vi "servertest.vi"() -> ()   [LabVIEW 2017]
uses:
  <vilib>/httpClient/ClientHandle.ctl
  <vilib>/httpClient/POSTBuffer.vi
  <vilib>/httpClient/LabVIEWHTTPClient.lvlib
panel:
  out "temp":i32
  out "element":T1
  out "value 2":T2
  in  "?":T3
  in  "url":string="getTC"
  out "body":string
  out "headers":string
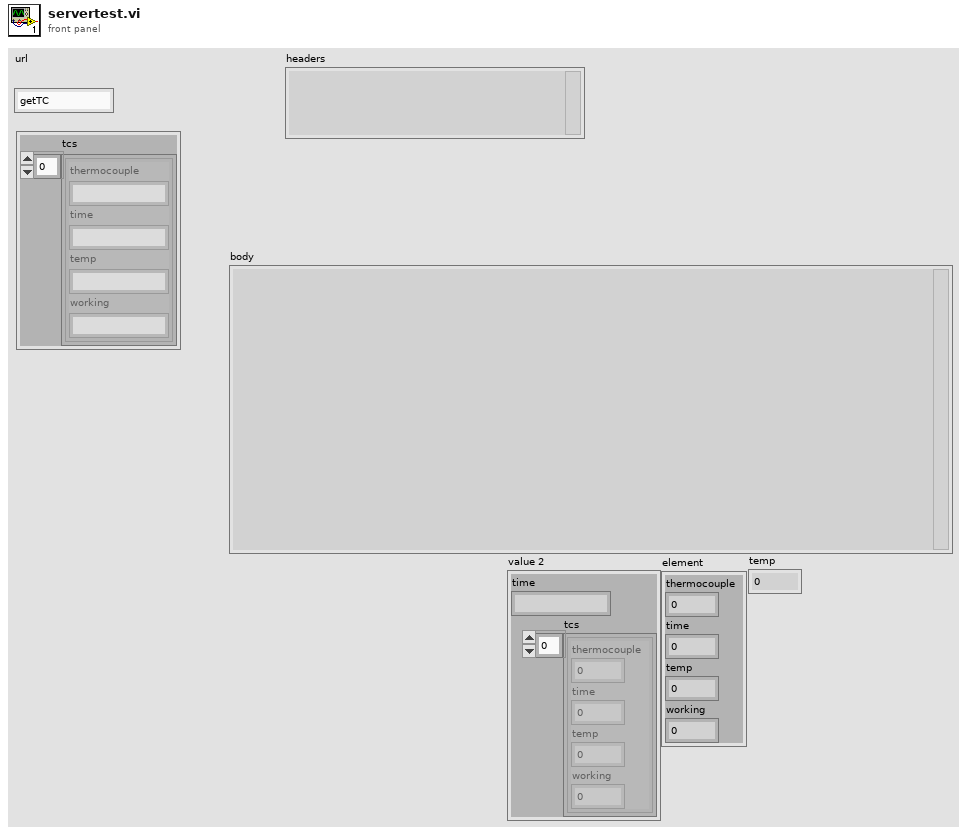
[diagram p1: front panel]
types:
  T1 = cluster{"thermocouple":i32, "time":i32, "temp":i32, "working":i32}
  T2 = cluster{"time":string, "tcs":cluster{"thermocouple":i32, "time":i32, "temp":i32, "working":i32}[]}
  T3 = cluster{"tcs":cluster{"thermocouple":string, "time":string, "temp":string, "working":string}[]}
  T4 = typedef "LabVIEWHTTPClient.lvlib/ClientHandle.ctl" = refnum<k1>
  T5 = cluster{"go":bool, "Http session":T4, "URL prefex":string}
  T6 = cluster{"thermocouple":i32, "time":i32, "temp":i32, "working":i32}[]
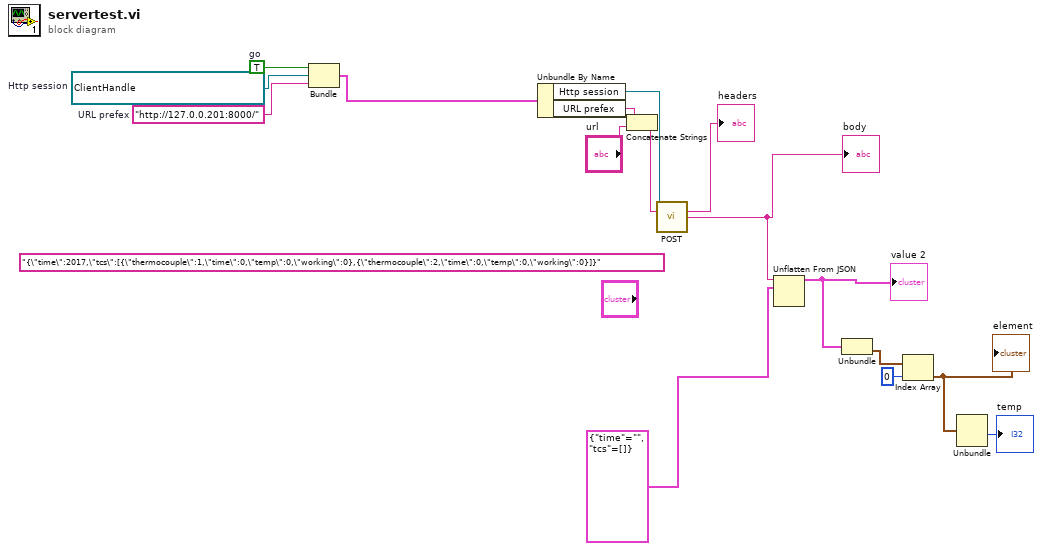
[diagram p0: block diagram]
diagram:
  (unwired) "{\"time\":2017,\"tcs\":[{\"thermocouple\":1,\"time\":0,\"temp\":0,\"working\":0},{\"thermocouple\":2,\"time\":0,\"temp\":0,\"working\":0}]}" ("JSON string")
  w14 = "http://127.0.0.201:8000/"  # URL prefex
  w15 = T4 refnum  # Http session
  w16 = TRUE  # go
  n1 = Bundle("go"=w16, "Http session"=w15, "URL prefex"=w14) -> (w9:T5)  [unwired: 1 in]
  n2 = Unbundle By Name(w9) -> ("Http session"=w13:T4, "URL prefex"=w11:string)
  n3 = Concatenate Strings(w11, "url") -> (w12:string)
  n4 = call-poly <vilib>:"POST.vi"("client handle"=w13, "url"=w12) -> ("headers"=→"headers":string, "body"=w7:string)  [unwired: 10 in, 2 out]
  "body" <- w7
  n5 = Unflatten From JSON(JSON string=w7, type and defaults=T2 {"time"="", "tcs"=[]}) -> (value=w5:T2)  [unwired: 5 in, 1 out]
  "value 2" <- w5
  n6 = Unbundle(w5) -> ("tcs"=w4:T6)  [unwired: 1 out]
  n7 = Index Array(array=w4, index=0) -> (element=w2:T1)
  "element" <- w2
  n8 = Unbundle(w2) -> ("temp"=→"temp":i32)  [unwired: 3 out]
